vi "Read_Bytes.vi"(6 "Queues":T1, 8 "Status/Errors in":refnum<vi>, 9 "Read bytes parameters":T3 {"Read bytes"."Max bytes read" format="%#.0f"}, 10 "Timer parameters":refnum<vi>, 11 "Devices":T2) -> ()   [LabVIEW 2010]
uses:
  Controls/Read_Bytes_Parameters.ctl
  Controls/Stop_Loop.ctl
  Controls/Read_Bytes.ctl
  Controls/Devices.ctl
  Controls/Queues.ctl
  Controls/One_Second.ctl
  Controls/GPS_Timestamp.ctl
  Controls/Status_Errors_Elements.ctl
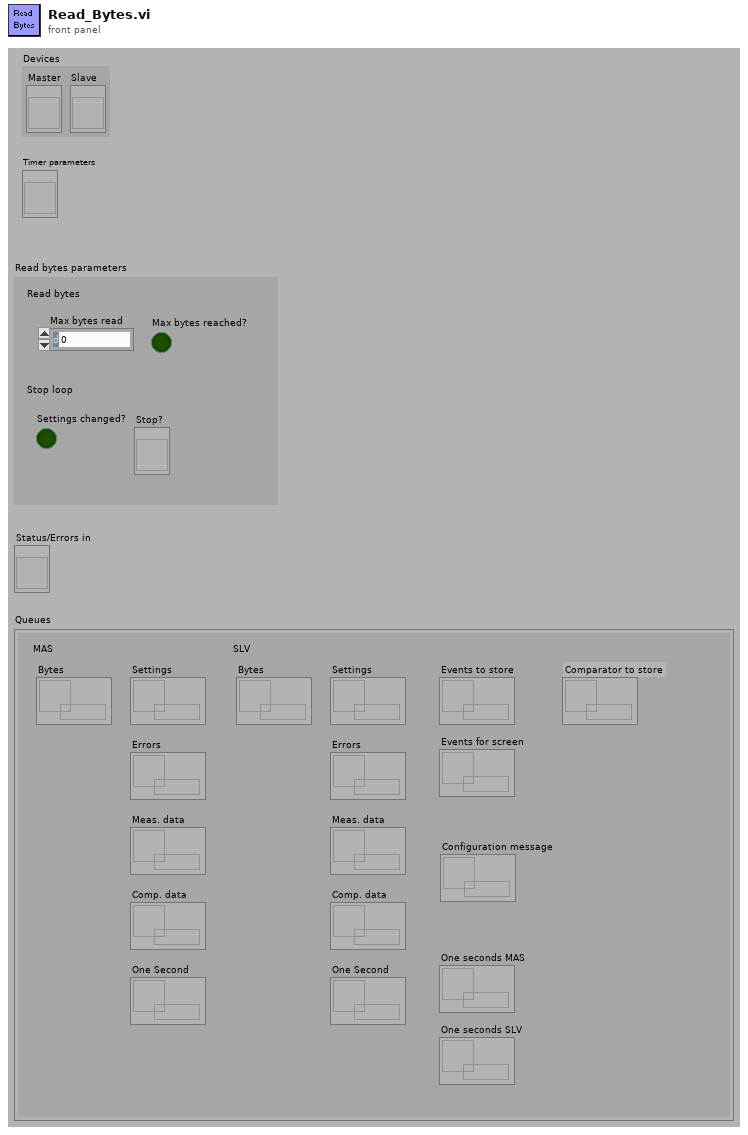
[diagram p1: front panel]
types:
  T1 = typedef "Queues.ctl" = cluster{"MAS":cluster{"Bytes":refnum<queue>, "Settings":refnum<queue>, "Errors":refnum<queue>, "Meas. data":refnum<queue>, "One Second":refnum<queue>, "Comp. data":refnum<queue>}, "SLV":cluster{"Bytes":refnum<queue>, "Settings":refnum<queue>, "Errors":refnum<queue>, "Meas. data":refnum<queue>, "One Second":refnum<queue>, "Comp. data":refnum<queue>}, "Events to store":refnum<queue>, "Events for screen":refnum<queue>, "One seconds MAS":refnum<queue>, "One seconds SLV":refnum<queue>, "Configuration message":refnum<queue>, "Comparator to store":refnum<queue>}
  T2 = typedef "Devices.ctl" = cluster{"Master":refnum<vi>, "Slave":refnum<vi>}
  T3 = typedef "Read_Bytes_Parameters.ctl" = cluster{"Stop loop":T4, "Read bytes":T5}
  T4 = typedef "Stop_Loop.ctl" = cluster{"Settings changed?":bool, "Stop?":refnum<vi>}
  T5 = typedef "Read_Bytes.ctl" = cluster{"Max bytes read":u32, "Max bytes reached?":bool}
  T6 = typedef "Status_Errors_Elements.ctl" = enum16{"Default", "Errors", "Master status", "Slave status", "Master connected?", "Slave connected?", "Master GPS on board?", "Slave GPS on board?", "Master: slave detected?", "Slave: slave detected?", "Last message from master", "Last message from slave", "Master temperature"}
  T7 = typedef "Command_Read_Bytes.ctl" = enum16{"Read", "Stop loop", "No action"}
  T8 = typedef "Rendezvous RefNum" = refnum<k1>
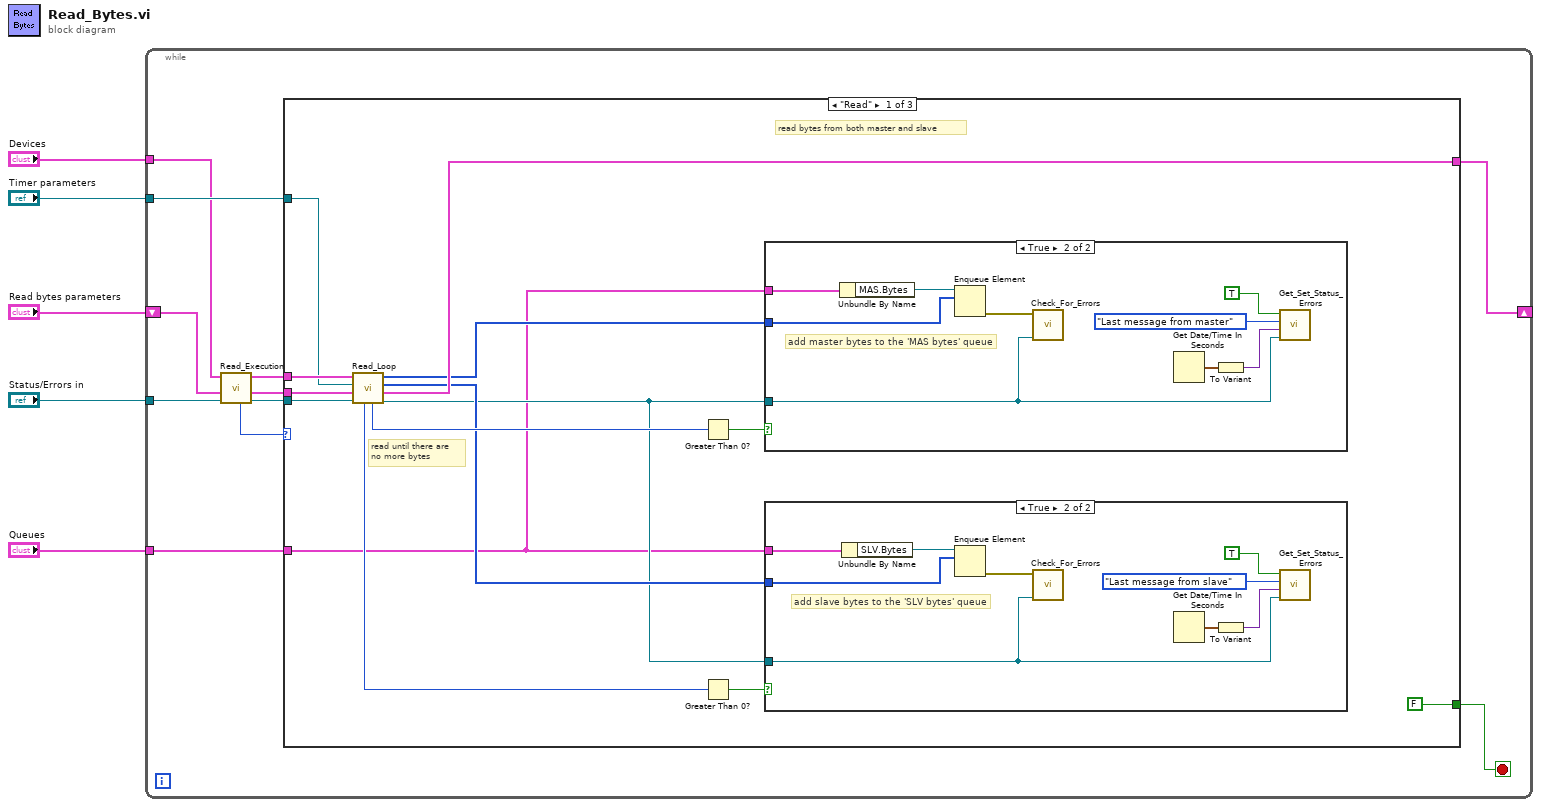
[diagram p0: block diagram]
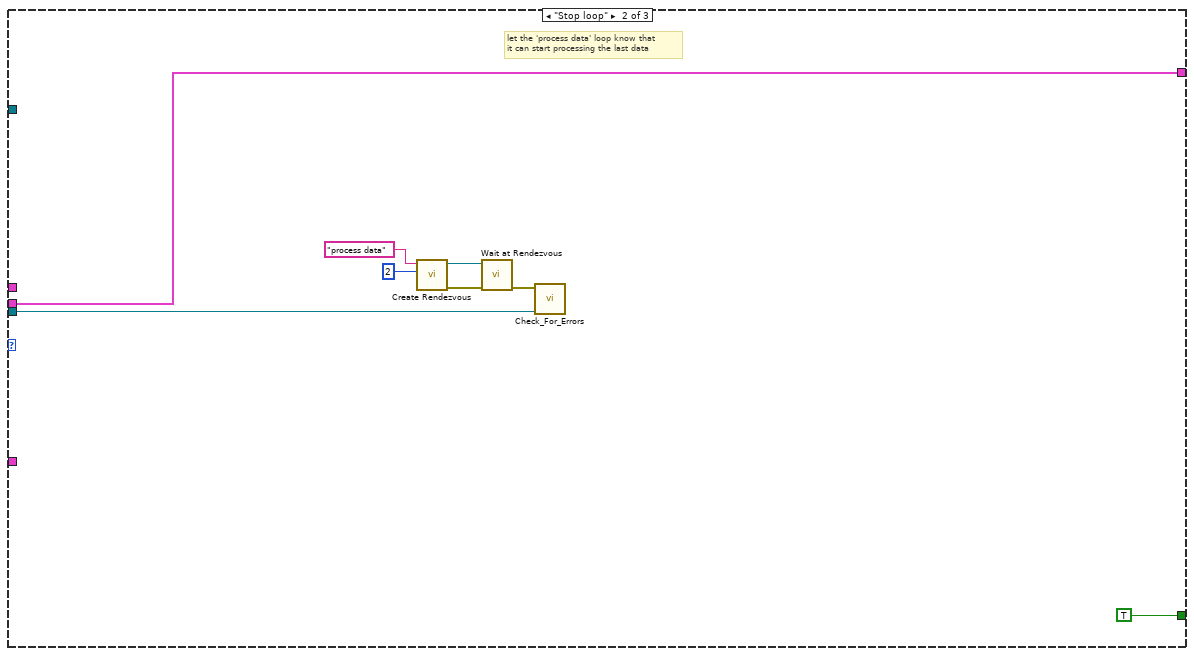
[diagram p4: hidden frame]
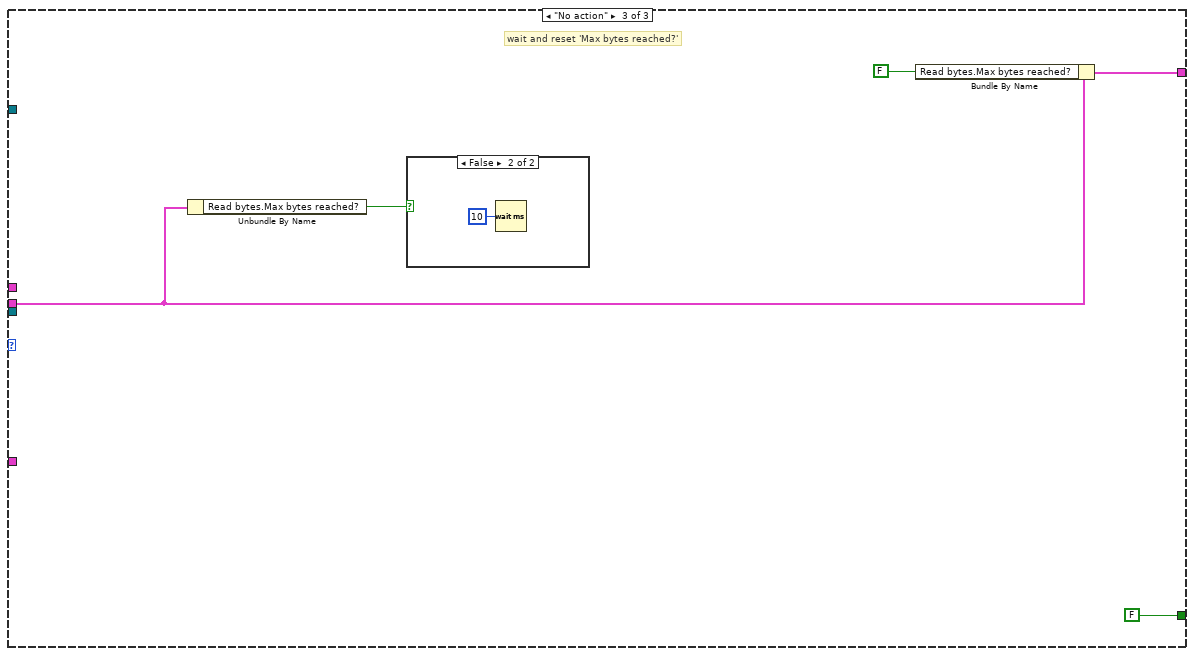
[diagram p5: hidden frame]
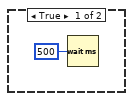
[diagram p6: hidden frame]
diagram:
  n1 = while {
    tunnel: "Devices" -> [w9]
    tunnel: "Status/Errors in" -> [w6]
    tunnel: "Queues" -> [w16]
    tunnel: "Timer parameters" -> [w15]
    shift-right: [w8] -> _
    shift-left: "Read bytes parameters" -> [w10]
    stop <- w14 stop-if-true
    n2 = call "Read_Execution.vi"("Status/Errors in"=w6, "Read bytes parameters in"=w10, "Devices in"=w9) -> ("Status/Errors out"=w13:refnum<vi>, "Read bytes parameters out"=w11:T3, "Devices out"=w12:T2, "Command"=w7:T7)  [unwired: 5 out]
    n3 = case shown="\"Read\"" w7 {
      tunnel: w12 -> [w29 _ _]
      tunnel: w11 -> [w28 w49 w58]
      tunnel: w13 -> [w30 w53 _]
      tunnel: w16 -> [w18 _ _]
      tunnel: w15 -> [w17 _ _]
      tunnel: [FALSE TRUE FALSE] -> w14
      tunnel: [w24 w49 w61] -> w8
      frame "Read" {
        # "read until there are\nno more bytes"
        # "read bytes from both master and slave"
        n4 = call "Read_Loop.vi"("Status/Errors in"=w30, "Read bytes parameters in"=w28, "Timer parameters"=w17, "Devices"=w29) -> ("Status/Errors out"=w20:refnum<vi>, "Read bytes parameters out"=w24:T3, "Slave bytes"=w22:u8[], "Master bytes"=w19:u8[], "# Master bytes"=w26:u32, "# Slave bytes"=w27:u32)  [unwired: 2 out]
        n5 = Greater Than 0?(x=w26) -> (x > 0?=w21:bool)
        n6 = Greater Than 0?(x=w27) -> (x > 0?=w23:bool)
        n7 = case shown="True" w21 {
          tunnel: w20 -> [_ w32]
          tunnel: w19 -> [_ w31]
          tunnel: w18 -> [_ w37]
          frame False {
          }
          frame True {
            # "add master bytes to the 'MAS bytes' queue"
            n8 = Unbundle By Name(w37) -> ("MAS.Bytes"=w39:refnum<queue>)
            n9 = Enqueue Element(queue=w39, element=w31) -> (error out=w38:errorcluster)  [unwired: 1 in, 3 out]
            n10 = call "Check_For_Errors.vi"("Status/Errors in"=w32, "error in"=w38) -> ()  [unwired: 10 out]
            n11 = Get Date/Time In Seconds() -> (seconds since 1Jan1904=w34:timestamp)
            n12 = To Variant(anything=w34) -> (Variant=w33:variant)
            n13 = call "Get_Set_Status_Errors.vi"("Status/Errors in"=w32, "Value in"=w33, "Element"=Status_Errors_Elements."Last message from master", "Set?"=TRUE) -> ()  [unwired: 8 out]
          }
        }
        n14 = case shown="True" w23 {
          tunnel: w20 -> [_ w40]
          tunnel: w22 -> [_ w41]
          tunnel: w18 -> [_ w46]
          frame False {
          }
          frame True {
            # "add slave bytes to the 'SLV bytes' queue"
            n15 = Unbundle By Name(w46) -> ("SLV.Bytes"=w48:refnum<queue>)
            n16 = Enqueue Element(queue=w48, element=w41) -> (error out=w47:errorcluster)  [unwired: 1 in, 3 out]
            n17 = call "Check_For_Errors.vi"("Status/Errors in"=w40, "error in"=w47) -> ()  [unwired: 10 out]
            n18 = Get Date/Time In Seconds() -> (seconds since 1Jan1904=w43:timestamp)
            n19 = To Variant(anything=w43) -> (Variant=w42:variant)
            n20 = call "Get_Set_Status_Errors.vi"("Status/Errors in"=w40, "Value in"=w42, "Element"=Status_Errors_Elements."Last message from slave", "Set?"=TRUE) -> ()  [unwired: 8 out]
          }
        }
      }
      frame "Stop loop" {
        # "let the 'process data' loop know that\nit can start processing the last data"
        n21 = call <vilib>:"Create Rendezvous.vi"("size (2)"=2, "name (unnamed)"="process data") -> ("error out"=w51:errorcluster, "rendezvous"=w54:T8)  [unwired: 1 in, 3 out]
        n22 = call <vilib>:"Wait at Rendezvous.vi"("error in (no error)"=w51, "rendezvous"=w54) -> ("error out"=w52:errorcluster)  [unwired: 1 in, 4 out]
        n23 = call "Check_For_Errors.vi"("Status/Errors in"=w53, "error in"=w52) -> ()  [unwired: 10 out]
      }
      frame "No action" {
        # "wait and reset 'Max bytes reached?'"
        n24 = Unbundle By Name(w58) -> ("Read bytes.Max bytes reached?"=w57:bool)
        n25 = case shown="False" w57 {
          frame True {
            n26 = Wait (ms)(milliseconds to wait=u32 500) -> ()  [unwired: 1 out]
          }
          frame False {
            n27 = Wait (ms)(milliseconds to wait=u32 10) -> ()  [unwired: 1 out]
          }
        }
        n28 = Bundle By Name(cluster=w58, "Read bytes.Max bytes reached?"=FALSE) -> (w61:T3)
      }
    }
  }
